vi "I2C Read.vi"(6 "Timeout ms (1000)":i32=1000, 7 "Slave Address (7-bit)":u8, 8 "Error In (No Error)":errorcluster, 9 "Keep Bus Busy":bool, 10 "Bytes to Read":u32, 11 "FPGA VI Reference In":T1) -> (0 "error out":errorcluster, 2 "Data Read":u8[](array[numeric]), 3 "FPGA VI Reference Out":T1)   [LabVIEW 2015]
uses:
  DSDB FPGA Ref.ctl
  <vilib>/rvi/errors/niLvFpgaAdjustHostInterfaceError.vi
  <vilib>/rvi/interface/nirviReadWriteControl/nirviReadWriteControl.xnode
  FPGA Bitfiles/Audio_FPGATarget_FPGAMain_3psOd07Wy8k.lvbitx
  FPGA Main.vi
  Sub VIs/Utilities/Start Boolean.ctl
  resource/NiAdept/NiAdept.dll
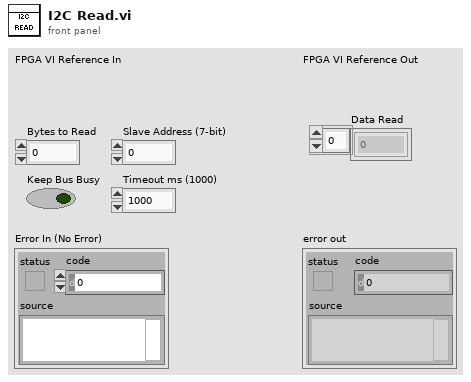
[diagram p1: front panel]
types:
  T1 = typedef "DSDB FPGA Ref.ctl" = refnum<k20>
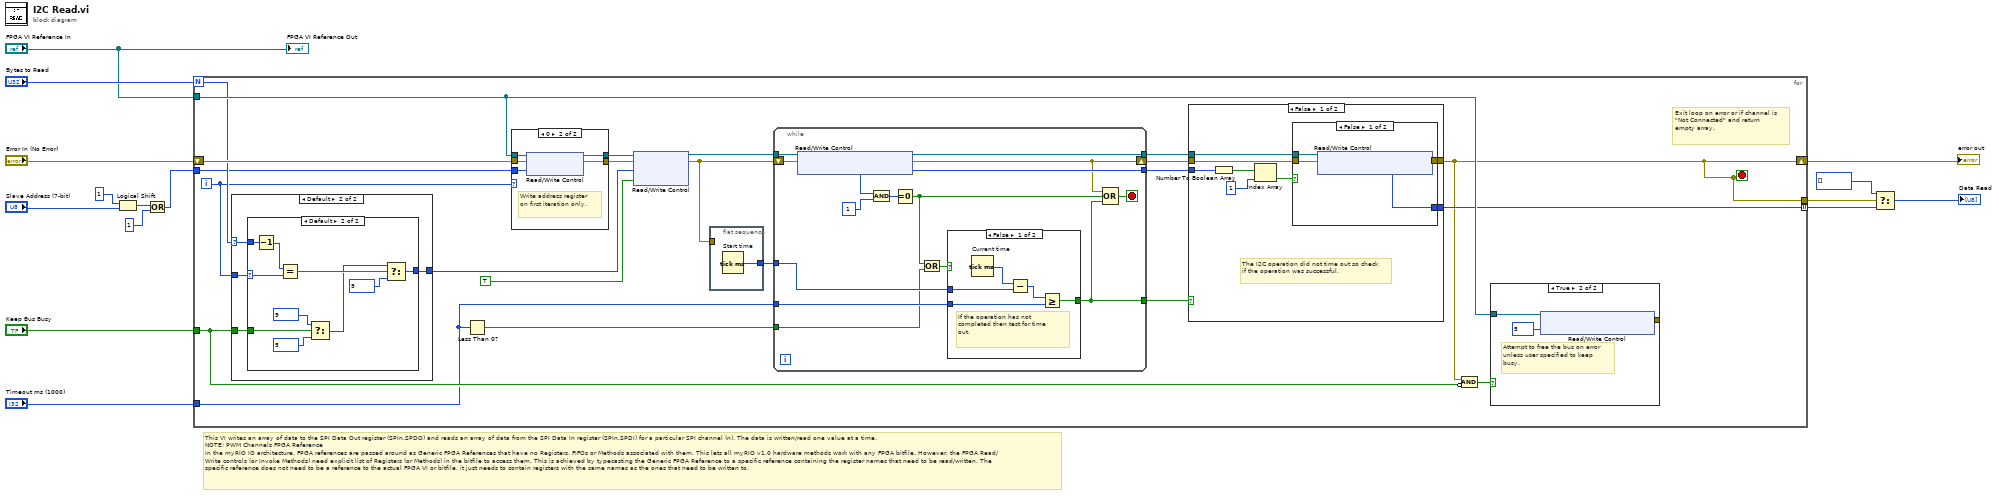
[diagram p0: block diagram]
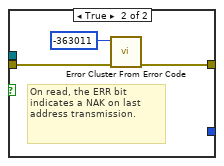
[diagram p2: hidden frame]
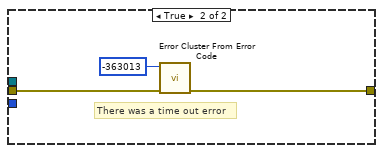
[diagram p3: hidden frame]
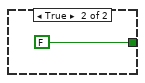
[diagram p6: hidden frame]
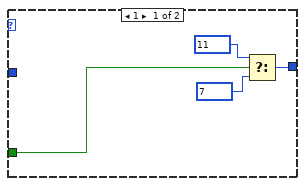
[diagram p7: hidden frame]
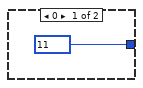
[diagram p8: hidden frame]
diagram:
  # "This VI writes an array of data to the SPI Data Out register (SPIn.SPDO) and reads an array of data from the SPI Data In register (SPIn.SPDI) for a particular SPI channel (n). The data is written/read one value at a time.\nNOTE: PWM Channels FPGA Reference\nIn the myRIO IO architecture, FPGA references are passed around as Generic FPGA References that have no Registers, FIFOs or Methods associated with them. This lets all myRIO v1.0 hardware methods work with any FPGA bitfile. However, the FPGA Read/Write controls (or Invoke Methods) need explicit list of Registers (or Methods) in the bitfile to access them. This is achieved by typecasting the Generic FPGA Reference to a specific reference containing the register names that need to be read/written. The specific reference does not need to be a reference to the actual FPGA VI or bitfile, it just needs to contain registers with the same names as the ones that need to be written to."
  n1 = Logical Shift(y=i8 1, x="Slave Address (7-bit)") -> (x << y=w13:u8)
  n2 = Or(x=w13, y=u8 1) -> (x .or. y?=w5:u8)
  n3 = for {
    N: "Bytes to Read" -> [w33]
    shift-right: [w16] -> w2
    shift-left: "Error In (No Error)" -> [w37]
    tunnel: "FPGA VI Reference In" -> [w36]
    tunnel: [w32] -> w7 mode=indexing
    tunnel: [w16] -> w8
    tunnel: "Keep Bus Busy" -> [w29]
    tunnel: w5 -> [w31]
    tunnel: "Timeout ms (1000)" -> [w28]
    i -> [w30]
    stop <- w16 stop-if-true
    # "Exit loop on error or if channel is \"Not Connected\" and return empty array."
    n4 = case shown="Default" w33 {
      selector: w33 -> [_ w92]
      tunnel: [w90 w93] -> w34
      tunnel: w30 -> [_ w94]
      tunnel: w29 -> [w88 w91]
      frame 1 {
        n5 = Select(t=u8 11 ("y"), s=w88, f=u8 7 ("y")) -> (s? t:f=w90:u8)
      }
      frame Default {
        n6 = case shown="Default" w94 {
          selector: w94 -> [_ w103]
          tunnel: [u8 11 ("y") w101] -> w93
          tunnel: w92 -> [_ w105]
          tunnel: w91 -> [_ w98]
          frame 0 {
          }
          frame Default {
            n7 = Decrement(x=w105) -> (x-1=w104:i32)
            n8 = Equal?(x=w104, y=w103) -> (x = y?=w102:bool)
            n9 = Select(t=u8 9 ("y"), s=w98, f=u8 5 ("y")) -> (s? t:f=w97:u8)
            n10 = Select(t=w97, s=w102, f=u8 9 ("y")) -> (s? t:f=w101:u8)
          }
        }
      }
    }
    n11 = Less Than 0?(x=w28) -> (x < 0?=w27:bool)
    n12 = case shown="0" w30 {
      tunnel: [w61 w66] -> w22
      tunnel: [w60 w65] -> w21
      tunnel: w36 -> [w61 w64]
      tunnel: w37 -> [w60 w63]
      tunnel: w31 -> [_ w62]
      frame Default {
      }
      frame 0 {
        # "Write address register on first iteration only."
        n13 = xnode "Read/Write Control"("FPGA VI Reference In"=w64, "error in"=w63, "I2C.Address"=w62) -> ("FPGA VI Reference Out"=w66:T1, "error out"=w65:errorcluster)
      }
    }
    n14 = xnode "Read/Write Control"("FPGA VI Reference In"=w22, "error in"=w21, "I2C.Control"=w34, "I2C.GO"=TRUE ("I2C0.GO")) -> ("FPGA VI Reference Out"=w26:T1, "error out"=w17:errorcluster)
    n15 = flat-sequence {
      tunnel: [w38] -> w19
      tunnel: w17 -> [_]
      frame #0 {
        n16 = Tick Count (ms) "Start time"() -> (millisecond timer value=w38:u32)
      }
    }
    n17 = while {
      tunnel: w26 -> [w79]
      shift-right: [w73] -> w25
      shift-left: w17 -> [w80]
      tunnel: [w75] -> w24
      tunnel: [w74] -> w23
      tunnel: w19 -> [w72]
      tunnel: [w71] -> w18
      tunnel: w28 -> [w70]
      tunnel: w27 -> [w68]
      stop <- w76 stop-if-true
      n18 = xnode "Read/Write Control"("FPGA VI Reference In"=w79, "error in"=w80) -> ("FPGA VI Reference Out"=w74:T1, "error out"=w73:errorcluster, "I2C.Status"=w75:u8)
      n19 = And(x=w75, y=u8 1) -> (x .and. y?=w77:u8)
      n20 = Equal To 0?(x=w77) -> (x = 0?=w67:bool)
      n21 = Or(x=w67, y=w68) -> (x .or. y?=w69:bool)
      n22 = case shown="False" w69 {
        tunnel: w72 -> [w83 _]
        tunnel: [w82 FALSE] -> w71
        tunnel: w70 -> [w81 _]
        frame False {
          # "If the operation has not completed then test for time out."
          n23 = Tick Count (ms) "Current time"() -> (millisecond timer value=w84:u32)
          n24 = Subtract(x=w84, y=w83) -> (x-y=w85:u32)
          n25 = Greater Or Equal?(x=w85, y=w81) -> (x >= y?=w82:bool)
        }
        frame True {
        }
      }
      n26 = Compound Arithmetic op=OR(w73, w67, w71) -> (w76:bool)
    }
    n27 = case shown="False" w18 {
      tunnel: w25 -> [w46 w55]
      tunnel: w24 -> [w45 _]
      tunnel: [w41 _] -> w32
      tunnel: w23 -> [w40 _]
      tunnel: [w39 w54] -> w16
      frame False {
        # "The I2C operation did not time out so check if the operation was successful."
        n28 = Number To Boolean Array(number=w45) -> (Boolean array=w44:bool[])
        n29 = Index Array(array=w44, index=1) -> (element=w43:bool)
        n30 = case shown="False" w43 {
          tunnel: w46 -> [w48 w51]
          tunnel: [w49 w53] -> w39
          tunnel: [w50 _] -> w41
          tunnel: w40 -> [w47 _]
          frame False {
            n31 = xnode "Read/Write Control"("FPGA VI Reference In"=w47, "error in"=w48) -> ("error out"=w49:errorcluster, "I2C.DataIn"=w50:u8)  [unwired: 1 out]
          }
          frame True {
            # "On read, the ERR bit indicates a NAK on last address transmission."
            n32 = call <vilib>:"Error Cluster From Error Code.vi"("error in (no error)"=w51, "error code (0)"=-363011) -> ("error out"=w53:errorcluster)  [unwired: 7 in]
          }
        }
      }
      frame True {
        # "There was a time out error"
        n33 = call <vilib>:"Error Cluster From Error Code.vi"("error in (no error)"=w55, "error code (0)"=-363013) -> ("error out"=w54:errorcluster)  [unwired: 7 in]
      }
    }
    n34 = Compound Arithmetic op=AND(w16, invert w29) -> (w20:bool)
    n35 = case shown="True" w20 {
      tunnel: w36 -> [_ w59]
      tunnel: [_ w57] -> _
      frame False {
      }
      frame True {
        # "Attempt to free the bus on error unless user specified to keep busy."
        n36 = xnode "Read/Write Control"("FPGA VI Reference In"=w59, "I2C.Control"=u8 5 ("I2C.C_0.CNTL")) -> ("error out"=w57:errorcluster)  [unwired: 1 in, 1 out]
      }
    }
  }
  "error out" <- w2
  n37 = Select(t=u8[] [], s=w8, f=w7) -> (s? t:f=→"Data Read":u8[])
  "FPGA VI Reference Out" <- "FPGA VI Reference In"
